vi "State_Machine.vi"(8 "error in (no error)":errorcluster caption="entrée d'erreur (pas d'erreur)", 11 "Get_Voltage en entrée":refnum<class "Read_Multimeter.lvclass">) -> (0 "error out":errorcluster caption="sortie d'erreur", 2 "Json_String":string, 3 "Get_Voltage en sortie":refnum<class "Read_Multimeter.lvclass">)   [LabVIEW 2020, in "Library Test.lvlib" / "Read_Multimeter.lvclass"]
uses:
  Read_Multimeter.lvclass
  C:/Users/ngarcin/OneDrive - Altyor/Standard TB/Class/Test/Test (Default)/Test (Default).lvclass
  JSON API/JSON Value/Set from JSON string.vi
  Instrument/Instrument (Default)/Class Instrument (Default).lvclass
  JSON API/JSON Value/JSON Value.lvclass
  Read_Multimeter.lvclass/Read_Multimeter.ctl
  JSON API/Variant JSON/Variant JSON.lvlib
  JSON API/Get Polymorphic/JSON GetSet.lvlib
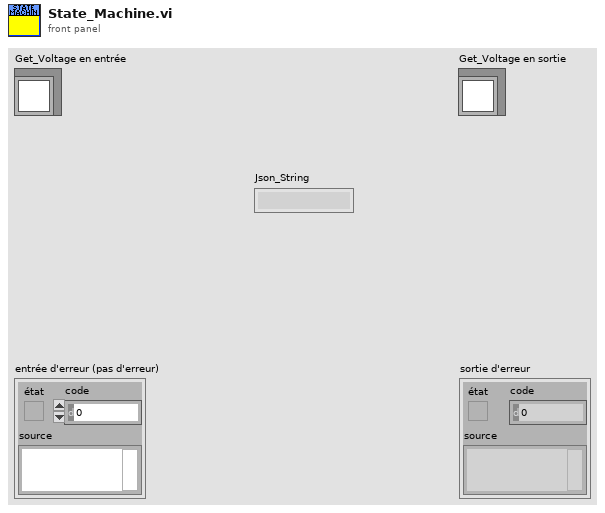
[diagram p1: front panel]
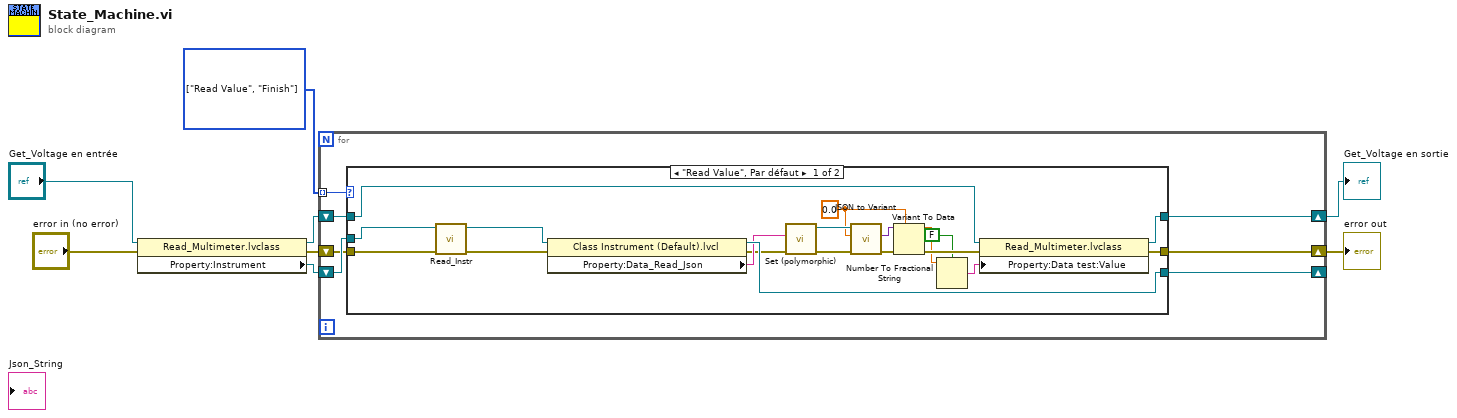
[diagram p0: block diagram]
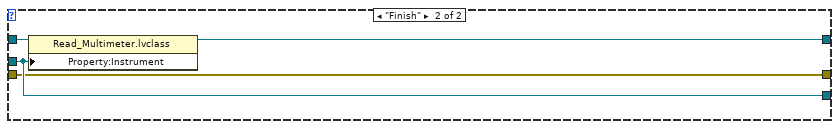
[diagram p2: hidden frame]
diagram:
  w7 = enum16{"Init", "Read Value", "Finish"}[] [enum."Read Value", enum."Finish"] items=["Init", "Read Value", "Finish"]
  n1 = property class="Read_Multimeter.lvclass"(reference="Get_Voltage en entrée", error in="error in (no error)") -> (reference out=w5:refnum<class "Read_Multimeter.lvclass">, error out=w1:errorcluster, "Property:Instrument"=w6:refnum<class "Class Instrument (Default).lvclass">)
  n2 = for {
    tunnel: w7 -> [w15] mode=indexing
    shift-right: [w13] -> _
    shift-left: w6 -> [w14]
    shift-right: [w11] -> w3
    shift-left: w5 -> [w12]
    shift-right: [w9] -> w4
    shift-left: w1 -> [w10]
    n3 = case shown="\"Read Value\", Par défaut" w15 {
      tunnel: w14 -> [w34 w36]
      tunnel: [w30 w36] -> w13
      tunnel: w12 -> [w32 w38]
      tunnel: [w17 w37] -> w11
      tunnel: w10 -> [w33 w35]
      tunnel: [w29 w35] -> w9
      frame "Read Value", Default {
        w20 = 0.0
        n4 = call-dynamic "Read_Instr.vi"("error in (no error)"=w33, "Class Instrument (Default) en entrée"=w34) -> ("error out"=w28:errorcluster, "Class Instrument (Default) en sortie"=w31:refnum<class "Class Instrument (Default).lvclass">)  [unwired: 8 in]
        n5 = property class="Class Instrument (Default).lvcl"(reference=w31, error in=w28) -> (reference out=w30:refnum<class "Class Instrument (Default).lvclass">, error out=w23:errorcluster, "Property:Data_Read_Json"=w24:string)
        n6 = call-poly "Set (polymorphic).vi"("error in (no error)"=w23, "JSON stream"=w24) -> ("error out"=w27:errorcluster, "JSON Value out"=w25:refnum<class "JSON Value.lvclass">)  [unwired: 7 in, 1 out]
        n7 = call "JSON to Variant.vi"("error in (no error)"=w27, "Variant (Data Type)"=w20, "JSON Value"=w25) -> ("error out"=w26:errorcluster, "Variant out"=w22:variant)  [unwired: 7 in]
        n8 = Variant To Data(error in=w26, type=w20, Variant=w22) -> (data=w19:dbl, error out=w21:errorcluster)
        n9 = Number To Fractional String(use system decimal point (T)=FALSE ("utiliser le séparateur décimal du système (V)"), number=w19) -> (F-format string=w18:string)  [unwired: 2 in]
        n10 = property class="Read_Multimeter.lvclass"(reference=w32, error in=w21, "Property:Data test:Value"=w18) -> (reference out=w17:refnum<class "Read_Multimeter.lvclass">, error out=w29:errorcluster)
      }
      frame "Finish" {
        n11 = property class="Read_Multimeter.lvclass"(reference=w38, "Property:Instrument"=w36) -> (reference out=w37:refnum<class "Read_Multimeter.lvclass">)  [unwired: 1 in, 1 out]
      }
    }
  }
  "error out" <- w4
  "Get_Voltage en sortie" <- w3
